vi "Async Loop Control.vi"(7 "Action":T17, 8 "error in (no error)":errorcluster, 10 "RT Data In":T1 {"Acyclic Frame Refs" format="%.0x"; "Label Transfer Config"."Block Data Refs"."Data Reference" format="%.0x"; "Status Config"."HWOut Dur Ref" format="%.0x"; "Status Config"."HWIn Dur Ref" format="%.0x"; "Status Config"."HWOut Count Ref" format="%.0x"; "Status Config"."HWIn Count Ref" format="%.0x"; "Status Config"."Error Data Ref" format="%.0x"; "HWOutput Channels"."Message Settings"."Driver Data"."First Word" min=8 max=31; "HWOutput Channels"."Message Settings"."Driver Data"."Num Bits" min=1 max=32; "HWOutput Channels"."Message Settings"."Driver Data"."Start Bit" min=8 max=31; "HWOutput Channels"."Message Settings"."Block Data Refs"."Data Reference" format="%.0x"; "HWInput Channels"."Message Settings"."Driver Data"."First Word" min=8 max=31; "HWInput Channels"."Message Settings"."Driver Data"."Num Bits" min=1 max=32; "HWInput Channels"."Message Settings"."Driver Data"."Start Bit" min=8 max=31; "HWInput Channels"."Message Settings"."Block Data Refs"."Data Reference" format="%.0x"}) -> (0 "error out":errorcluster, 2 "RT Data Out":T1 {"Acyclic Frame Refs" format="%.0x"; "Label Transfer Config"."Block Data Refs"."Data Reference" format="%.0x"; "Status Config"."HWOut Dur Ref" format="%.0x"; "Status Config"."HWIn Dur Ref" format="%.0x"; "Status Config"."HWOut Count Ref" format="%.0x"; "Status Config"."HWIn Count Ref" format="%.0x"; "Status Config"."Error Data Ref" format="%.0x"; "HWOutput Channels"."Message Settings"."Driver Data"."First Word" min=8 max=31; "HWOutput Channels"."Message Settings"."Driver Data"."Num Bits" min=1 max=32; "HWOutput Channels"."Message Settings"."Driver Data"."Start Bit" min=8 max=31; "HWOutput Channels"."Message Settings"."Block Data Refs"."Data Reference" format="%.0x"; "HWInput Channels"."Message Settings"."Driver Data"."First Word" min=8 max=31; "HWInput Channels"."Message Settings"."Driver Data"."Num Bits" min=1 max=32; "HWInput Channels"."Message Settings"."Driver Data"."Start Bit" min=8 max=31; "HWInput Channels"."Message Settings"."Block Data Refs"."Data Reference" format="%.0x"})   [LabVIEW 2013, in "AIT 1553 Custom Device.lvlib"]
doc: "Controls the Async Loops (Meas Write/Read, Char Write/Read) according to the action input."
uses:
  AIT 1553 Custom Device.lvlib
  RT Controls/AIT 1553  - RT Data.ctl
  RT Controls/AIT 1553 - RT HW Channel.ctl
  RT Controls/AIT 1553 - Bus Section.ctl
  RT Controls/AIT 1553 - RT Message Settings.ctl
  <vilib>/NI Veristand/Custom Device API/Block Data Reference.ctl
  <vilib>/NI Veristand/Custom Device API/Data Reference.ctl
  RT Controls/AIT 1553 - Driver Data.ctl
  Controls and Global/Start Bit.ctl
  Controls and Global/Number of Bits.ctl
  RT Controls/AIT 1553 - Board Config Info.ctl
  RT Controls/AIT 1553 - Hardware Type.ctl
  RT Controls/Error Qs.ctl
  RT Controls/Status Channels Config.ctl
  RT Controls/FIFO.ctl
  RT Controls/Label Transfer Config.ctl
  <vilib>/NI Veristand/Custom Device API/Custom Device Item Ref.ctl
  RT Controls/Async Loop Control Enum.ctl
  <vilib>/NI Veristand/Custom Device API/Custom Device API.lvlib
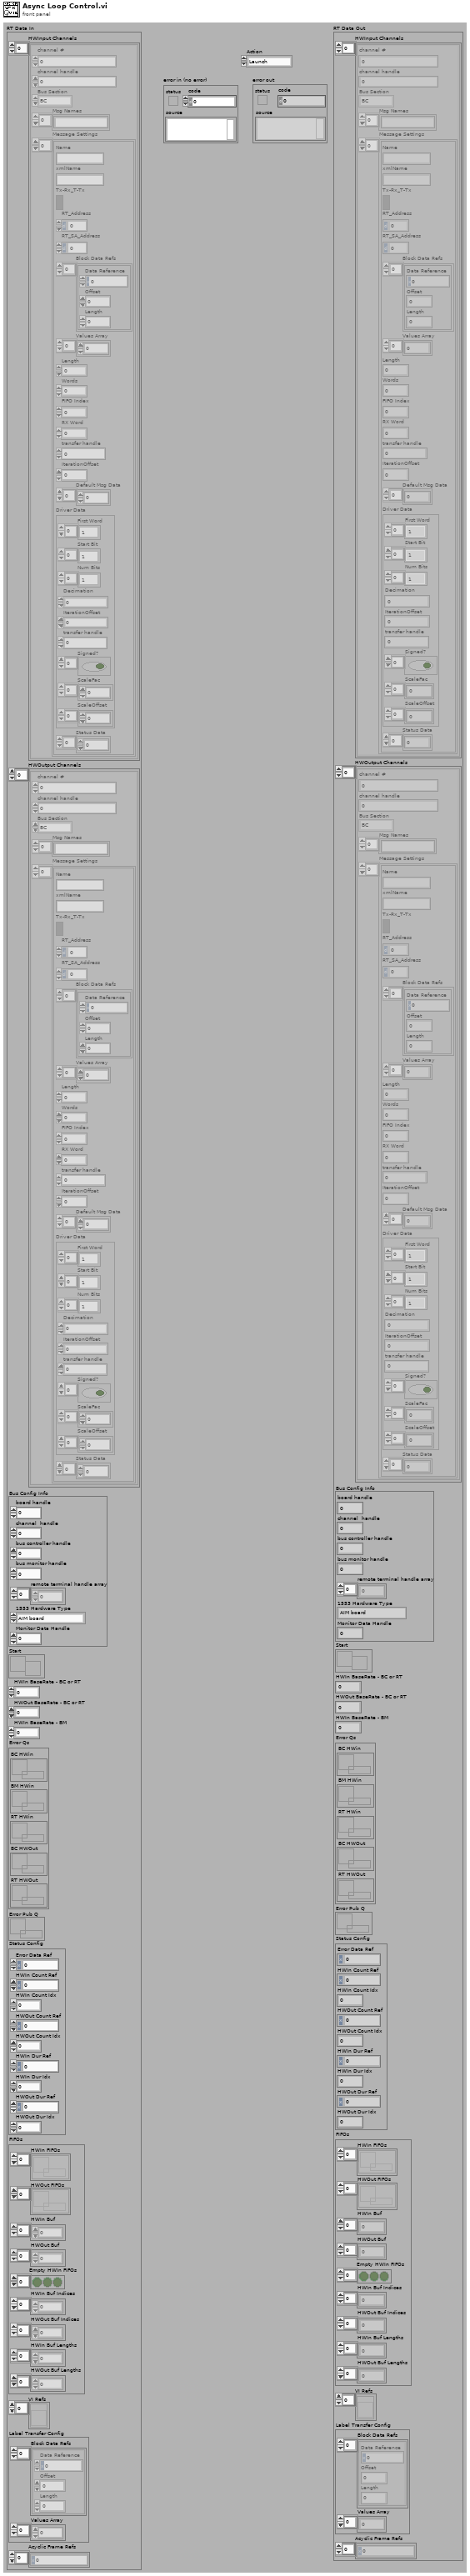
[diagram p1: front panel]
types:
  T1 = typedef "AIT 1553 Custom Device.lvlib/AIT 1553  - RT Data.ctl" = cluster{"HWInput Channels":T2[], "HWOutput Channels":T2[], "Bus Config Info":T10, "Start":refnum<notifier>, "HWIn BaseRate - BC or RT":i64, "HWOut BaseRate - BC or RT":i64, "HWIn BaseRate - BM":i64, "Error Qs":T12, "Error Pub Q":refnum<queue>, "Status Config":T13, "FIFOs":T14, "VI Refs":refnum<vi>[], "Label Transfer Config":T15, "Acyclic Frame Refs":T16[]}
  T2 = typedef "AIT 1553 Custom Device.lvlib/AIT 1553 - RT HW Channel.ctl" = cluster{"channel #":u16, "channel handle":u32, "Bus Section":T3, "Msg Names":string[], "Message Settings":T4[]}
  T3 = typedef "AIT 1553 Custom Device.lvlib/AIT 1553 - Bus Section.ctl" = enum16{"BC", "BM", "RT"}
  T4 = typedef "AIT 1553 Custom Device.lvlib/AIT 1553 - RT Message Settings.ctl" = cluster{"Name":string, "xmlName":string, "Tx-Rx_T-Tx":bool, "RT_Address":u8, "RT_SA_Address":u8, "Block Data Refs":T5[], "Values Array":dbl[], "Length":i32, "Words":i32, "FIFO Index":i32, "RX Word":u32, "transfer handle":u32, "IterationOffset":i32, "Default Msg Data":u16[], "Driver Data":T7, "Status Data":u32[]}
  T5 = typedef "Custom Device API.lvlib/Block Data Reference.ctl" = cluster{"Data Reference":T6, "Offset":i32, "Length":i32}
  T6 = typedef "Custom Device API.lvlib/Data Reference.ctl" = i32
  T7 = typedef "AIT 1553 Custom Device.lvlib/AIT 1553 - Driver Data.ctl" = cluster{"First Word":T8[], "Start Bit":T8[], "Num Bits":T9[], "Decimation":i32, "IterationOffset":i32, "transfer handle":u32, "Signed?":bool[], "ScaleFac":dbl[], "ScaleOffset":dbl[]}
  T8 = typedef "AIT 1553 Custom Device.lvlib/Start Bit.ctl" = i32
  T9 = typedef "AIT 1553 Custom Device.lvlib/Number of Bits.ctl" = i32
  T10 = typedef "AIT 1553 Custom Device.lvlib/AIT 1553 - Board Config Info.ctl" = cluster{"board handle":u32, "channel  handle":u32, "bus controller handle":u32, "bus monitor handle":u32, "remote terminal handle array":u32[], "1553 Hardware Type":T11, "Monitor Data Handle":u32}
  T11 = typedef "AIT 1553 Custom Device.lvlib/AIT 1553 - Hardware Type.ctl" = enum16{"AIM board", "AIT Board"}
  T12 = typedef "AIT 1553 Custom Device.lvlib/Error Qs.ctl" = cluster{"BC HWin":refnum<queue>, "BM HWin":refnum<queue>, "RT HWin":refnum<queue>, "BC HWOut":refnum<queue>, "RT HWOut":refnum<queue>}
  T13 = typedef "AIT 1553 Custom Device.lvlib/Status Channels Config.ctl" = cluster{"Error Data Ref":T6, "HWIn Count Ref":T6, "HWIn Count Idx":i32, "HWOut Count Ref":T6, "HWOut Count Idx":i32, "HWIn Dur Ref":T6, "HWIn Dur Idx":i32, "HWOut Dur Ref":T6, "HWOut Dur Idx":i32}
  T14 = typedef "AIT 1553 Custom Device.lvlib/FIFO.ctl" = cluster{"HWIn FIFOs":refnum<k33>[], "HWOut FIFOs":refnum<k33>[], "HWIn Buf":dbl[], "HWOut Buf":dbl[], "Empty HWIn FIFOs":bool[], "HWIn Buf Indices":i32[], "HWOut Buf Indices":i32[], "HWIn Buf Lengths":i32[], "HWOut Buf Lengths":i32[]}
  T15 = typedef "AIT 1553 Custom Device.lvlib/Label Transfer Config.ctl" = cluster{"Block Data Refs":T5[], "Values Array":dbl[]}
  T16 = typedef "Custom Device API.lvlib/Custom Device Item Ref.ctl" = u64
  T17 = typedef "AIT 1553 Custom Device.lvlib/Async Loop Control Enum.ctl" = enum16{"Launch", "Start", "Stop"}
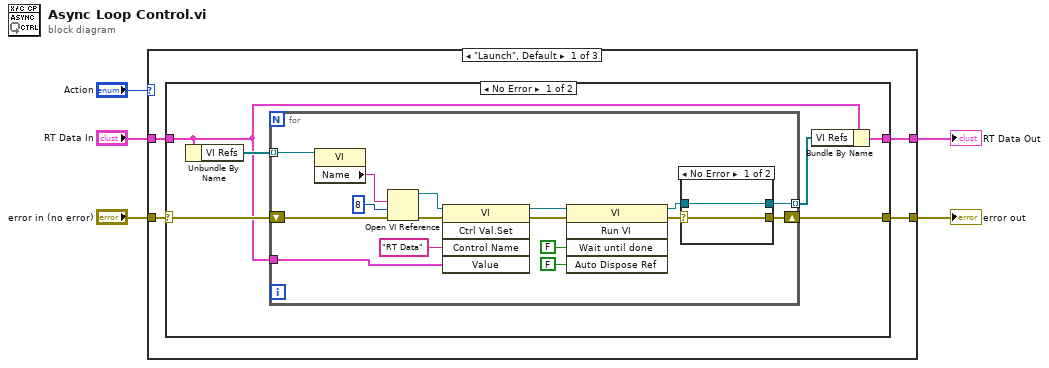
[diagram p0: block diagram]
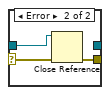
[diagram p2: hidden frame]
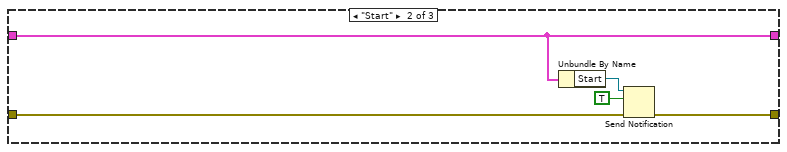
[diagram p4: hidden frame]
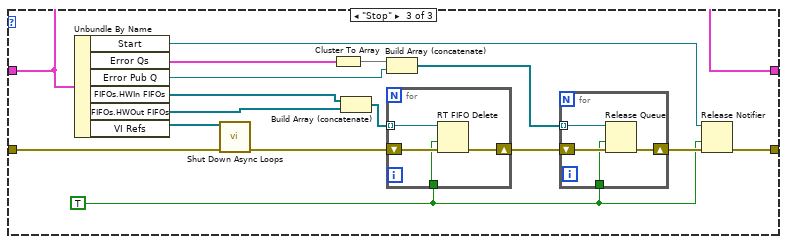
[diagram p5: hidden frame]
diagram:
  n1 = case shown="\"Launch\", Default" "Action" {
    tunnel: [w9 w40 w51] -> w5
    tunnel: "error in (no error)" -> [w8 w42 w46]
    tunnel: "RT Data In" -> [w7 w39 w49]
    tunnel: [w6 w39 w49] -> w1
    frame "Launch", Default {
      n2 = case shown="No Error" w8 {
        selector: w8 -> [w15 w38]
        tunnel: [w14 w38] -> w9
        tunnel: w7 -> [w10 w37]
        tunnel: [w11 w37] -> w6
        frame No Error {
          n3 = Unbundle By Name(w10) -> ("VI Refs"=w13:refnum<vi>[])
          n4 = for {
            shift-right: [w28] -> w14
            shift-left: w15 -> [w31]
            tunnel: w13 -> [w30] mode=indexing
            tunnel: w10 -> [w16]
            tunnel: [w29] -> w12 mode=indexing
            n5 = property class="VI"(reference=w30) -> ("Name"=w27:string)  [unwired: 1 in, 2 out]
            n6 = Open VI Reference(vi path=w27, options=8, error in (no error)=w31) -> (vi reference=w19:refnum<vi>, error out=w20:errorcluster)  [unwired: 3 out]
            n7 = invoke class="VI" method="Ctrl Val.Set"(reference=w19, error in=w20, "Control Name"="RT Data", "Value"=w16) -> (reference out=w21:refnum<vi>, error out=w17:errorcluster)  [unwired: 1 in, 3 out]
            n8 = invoke class="VI" method="Run VI"(reference=w21, error in=w17, "Wait until done"=FALSE ("Wait Until Done"), "Auto Dispose Ref"=FALSE ("Auto Dispose Reference")) -> (reference out=w22:refnum<vi>, error out=w23:errorcluster)  [unwired: 1 in, 3 out]
            n9 = case shown="No Error" w23 {
              selector: w23 -> [w33 w36]
              tunnel: w22 -> [w32 w35]
              tunnel: [w33 w34] -> w28
              tunnel: [w32 _] -> w29
              frame No Error {
              }
              frame Error {
                n10 = Close Reference(reference=w35, error in (no error)=w36) -> (error out=w34:errorcluster)
              }
            }
          }
          n11 = Bundle By Name(cluster=w10, "VI Refs"=w12) -> (w11:T1)
        }
        frame Error {
        }
      }
    }
    frame "Start" {
      n12 = Unbundle By Name(w39) -> ("Start"=w43:refnum<notifier>)
      n13 = Send Notification(notification=TRUE, notifier=w43, error in (no error)=w42) -> (error out=w40:errorcluster)  [unwired: 1 out]
    }
    frame "Stop" {
      w50 = TRUE ("force destroy? (F)")
      n14 = Unbundle By Name(w49) -> ("Start"=w55:refnum<notifier>, "Error Qs"=w59:T12, "Error Pub Q"=w57:refnum<queue>, "FIFOs.HWIn FIFOs"=w54:refnum<k33>[], "FIFOs.HWOut FIFOs"=w47:refnum<k33>[], "VI Refs"=w44:refnum<vi>[])
      n15 = call "Shut Down Async Loops.vi"("VI Refs"=w44, "error in (no error)"=w46) -> ("error out"=w45:errorcluster)  [unwired: 13 in]
      n16 = Cluster To Array(cluster=w59) -> (array=w58:refnum<queue>[])
      n17 = Build Array (concatenate)(w54, w47) -> (w53:refnum<k33>[])
      n18 = Build Array (concatenate)(w58, w57) -> (w48:refnum<queue>[])
      n19 = for {
        shift-right: [w62] -> w52
        shift-left: w45 -> [w63]
        tunnel: w53 -> [w61] mode=indexing
        tunnel: w50 -> [w60]
        n20 = RT FIFO Delete(0:w61, 2:w60, 3:w63) -> (11:w62:errorcluster)
      }
      n21 = for {
        shift-right: [w66] -> w56
        shift-left: w52 -> [w67]
        tunnel: w48 -> [w65] mode=indexing
        tunnel: w50 -> [w64]
        n22 = Release Queue(queue=w65, force destroy? (F)=w64, error in (no error)=w67) -> (error out=w66:errorcluster)  [unwired: 2 out]
      }
      n23 = Release Notifier(notifier=w55, force destroy? (F)=w50, error in (no error)=w56) -> (error out=w51:errorcluster)  [unwired: 2 out]
    }
  }
  "error out" <- w5
  "RT Data Out" <- w1
